vi "Define_Crossconnection_Problem_by_Points_Indicies-1.vi"(6 "[IN] Track group":T1, 7 "[IN] Index of connected points \nwith initial point inside the track":i32[](array[numeric]), 8 "[IN] Index of connected tra\ncks with initial problem point":i32[](array[numeric]), 9 "[IN] Index of connected points \nwith other point inside the track":i32[](array[numeric]), 10 "[IN] Index of connected trac\nks with other problem point":i32[](array[numeric])) -> (1 "[OUT] Index in array for \nother problem \"111\" point":i32, 2 "[OUT] Index in array for \ninitial problem \"111\" point":i32, 3 "[OUT] The other point \nfor crossconnection found":bool)   [LabVIEW 2013]
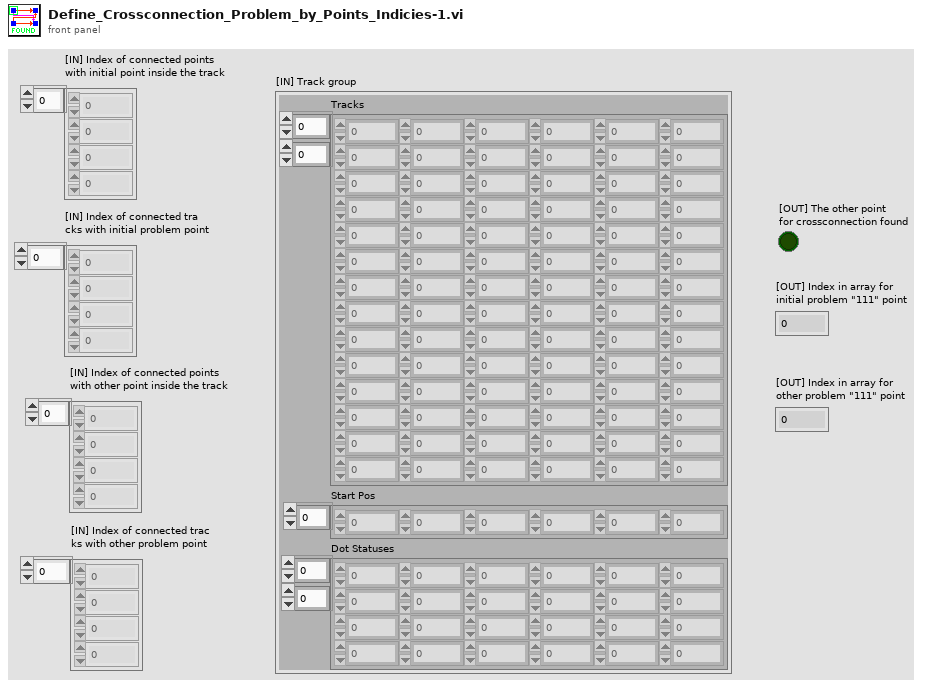
[diagram p1: front panel]
types:
  T1 = cluster{"Tracks":dbl[][], "Start Pos":i32[], "Dot Statuses":i16[][]}
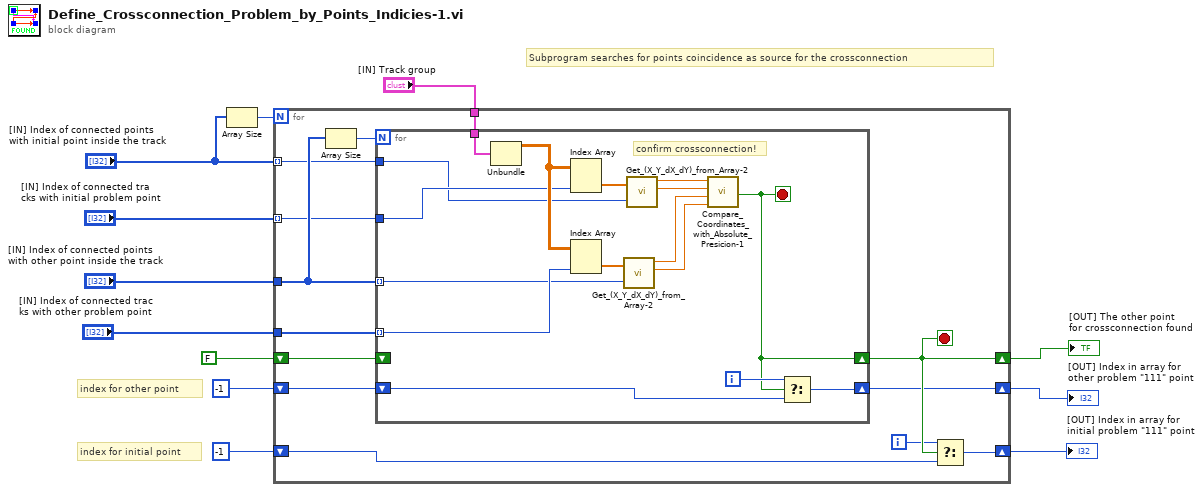
[diagram p0: block diagram]
diagram:
  # "index for initial point"
  # "index for other point"
  # "Subprogram searches for points coincidence as source for the crossconnection"
  n1 = Array Size(array="[IN] Index of connected points \nwith initial point inside the track") -> (size(s)=w12:i32)
  n2 = for {
    N: w12 -> [_]
    tunnel: "[IN] Index of connected points \nwith initial point inside the track" -> [w21] mode=indexing
    tunnel: "[IN] Index of connected tra\ncks with initial problem point" -> [w20] mode=indexing
    tunnel: "[IN] Index of connected points \nwith other point inside the track" -> [w24]
    tunnel: "[IN] Index of connected trac\nks with other problem point" -> [w23]
    shift-right: [w18] -> w6
    shift-left: FALSE -> [w22]
    shift-right: [w14] -> w3
    shift-left: -1 -> [w19]
    shift-right: [w15] -> w2
    shift-left: -1 -> [w16]
    tunnel: "[IN] Track group" -> [w13]
    i -> [w17]
    stop <- w18 stop-if-true
    n3 = Array Size(array=w24) -> (size(s)=w25:i32)
    n4 = for {
      N: w25 -> [_]
      tunnel: w24 -> [w31] mode=indexing
      tunnel: w23 -> [w35] mode=indexing
      shift-right: [w26] -> w18
      shift-left: w22 -> [_]
      tunnel: w21 -> [w33]
      tunnel: w20 -> [w36]
      shift-right: [w39] -> w14
      shift-left: w19 -> [w41]
      tunnel: w13 -> [w38]
      i -> [w40]
      stop <- w26 stop-if-true
      # "confirm crossconnection!"
      n5 = Unbundle(w38) -> ("Tracks"=w37:dbl[][])  [unwired: 2 out]
      n6 = Index Array(array=w37, index (col)=w36) -> (element=w34:dbl[])  [unwired: 1 in]
      n7 = Index Array(array=w37, index (col)=w35) -> (element=w32:dbl[])  [unwired: 1 in]
      n8 = call "Get_(X_Y_dX_dY)_from_Array-2.vi"("(X,Y,dX,dY)"=w32, "Index of Displacement"=w31) -> ("X"=w28:dbl, "Y"=w27:dbl)  [unwired: 2 out]
      n9 = call "Get_(X_Y_dX_dY)_from_Array-2.vi"("(X,Y,dX,dY)"=w34, "Index of Displacement"=w33) -> ("X"=w30:dbl, "Y"=w29:dbl)  [unwired: 2 out]
      n10 = call "Compare_Coordinates_with_Absolute_Presicion-1.vi"("X 1"=w30, "Y 1"=w29, "X 2"=w28, "Y 2"=w27) -> ("[OUT] Same coordinates?"=w26:bool)  [unwired: 1 in]
      n11 = Select(t=w40, s=w26, f=w41) -> (s? t:f=w39:i32)
    }
    n12 = Select(t=w17, s=w18, f=w16) -> (s? t:f=w15:i32)
  }
  "[OUT] The other point \nfor crossconnection found" <- w6
  "[OUT] Index in array for \nother problem \"111\" point" <- w3
  "[OUT] Index in array for \ninitial problem \"111\" point" <- w2
